vi "Parse Tag.vi"(8 "error in (no error)":errorcluster, 10 "Flattened Linked List":string, 11 "XML in":refnum<class "XML.lvclass">) -> (0 "error out":errorcluster, 1 "Tag":string, 2 "Flattened Linked List After Tag":string, 3 "XML out":refnum<class "XML.lvclass">, 4 "Nothing Found":bool, 5 "Ignore":bool, 6 "<Tag/>":bool)   [LabVIEW 2020, in "XML.lvlib" / "XML.lvclass"]
uses:
  <vilib>/gpm_packages/@cs/persistence/source/XML/XML.lvclass
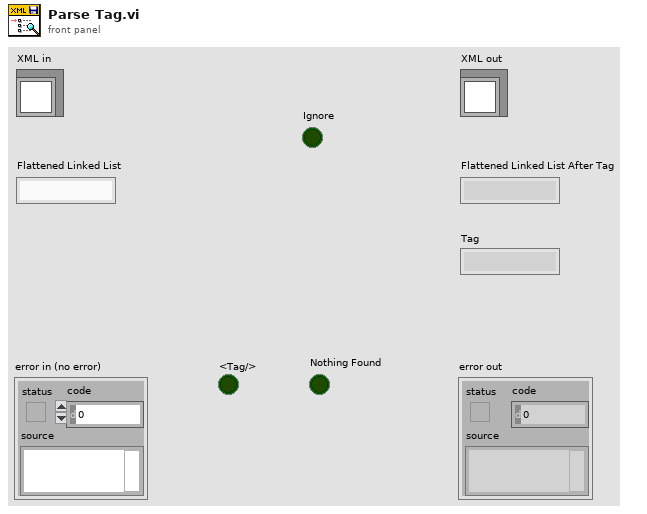
[diagram p1: front panel]
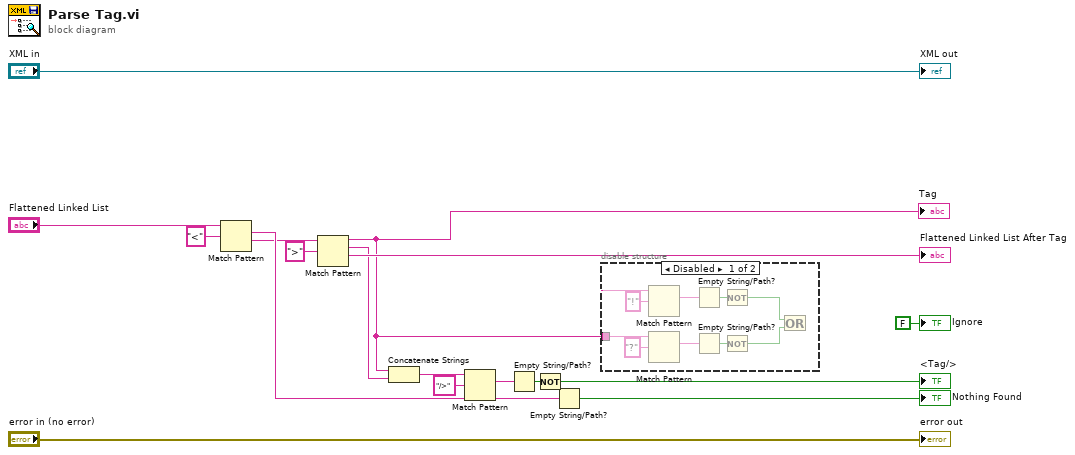
[diagram p0: block diagram]
diagram:
  n1 = Match Pattern(string="Flattened Linked List", regular expression="<") -> (match substring=w9:string, after substring=w4:string)  [unwired: 1 in, 2 out]
  n2 = Match Pattern(string=w4, regular expression=">") -> (before substring=w12:string, match substring=w3:string, after substring=→"Flattened Linked List After Tag":string)  [unwired: 1 in, 1 out]
  "Tag" <- w12
  n3 = Concatenate Strings(w12, w3) -> (w5:string)
  n4 = Match Pattern(string=w5, regular expression="/>") -> (match substring=w7:string)  [unwired: 1 in, 3 out]
  n5 = Empty String/Path?(string/path=w7) -> (empty?=w6:bool)
  n6 = Not(x=w6) -> (.not. x?=→"<Tag/>":bool)
  n7 = Empty String/Path?(string/path=w9) -> (empty?=→"Nothing Found":bool)
  n8 = disable-structure shown="Disabled" {
    disable-tunnel: w12 -> [w26 _]
    frame Disabled {
      n9 = Match Pattern(string=w26, regular expression="!") -> (match substring=w21:string)  [unwired: 1 in, 3 out]
      n10 = Match Pattern(string=w26, regular expression="?") -> (match substring=w24:string)  [unwired: 1 in, 3 out]
      n11 = Empty String/Path?(string/path=w21) -> (empty?=w22:bool)
      n12 = Empty String/Path?(string/path=w24) -> (empty?=w23:bool)
      n13 = Not(x=w22) -> (.not. x?=w18:bool)
      n14 = Not(x=w23) -> (.not. x?=w19:bool)
      n15 = Or(x=w18, y=w19) -> ()  [unwired: 1 out]
    }
    frame Enabled {
    }
  }
  "error out" <- "error in (no error)"
  "XML out" <- "XML in"
  "Ignore" <- FALSE ("Ignore")
